vi "Create Evaluations.vi"(8 "error in (no error)":errorcluster, 11 "IEvaluation in":refnum<class "Null Adapter.lvclass">) -> (0 "error out":errorcluster, 2 "Evaluations Out":T1[](array[typedef]) {"Low Limit" format="%#_13g"; "SI Scaling" items=["femto"=-15, "pico"=-12, "nano"=-9, "micro"=-6, "milli"=-3, "percent"=-2, ""=0, "kilo"=3, "mega"=6, "giga"=9, "tera"=12]}, 3 "IEvaluation out":refnum<class "Null Adapter.lvclass">)   [LabVIEW 2018, in "SeqAuto Evaluations.lvlib" / "Null Adapter.lvclass"]
uses:
  Null Adapter.lvclass
  C:/Sequence Automation/Plugins/SeqAuto IEvaluation.lvlibp/SeqAuto IEvaluation.lvclass
  Plugins/TestStand API Tools (TSAT).lvlibp/Evaluation Actions/Includes/Controls/TSAT Evaluation.ctl
  Plugins/TestStand API Tools (TSAT).lvlibp/Evaluation Actions/Includes/Controls/TSAT Eval SI Unit Scaling.ctl
  Plugins/TestStand API Tools (TSAT).lvlibp/Evaluation Actions/Includes/Controls/TSAT Evaluation Type.ctl
  Plugins/SeqAuto IEvaluation.lvlibp/Read Measurement Name.vi
  Plugins/TestStand API Tools (TSAT).lvlibp/Evaluation Actions/TSAT Evaluation Actions.lvlib
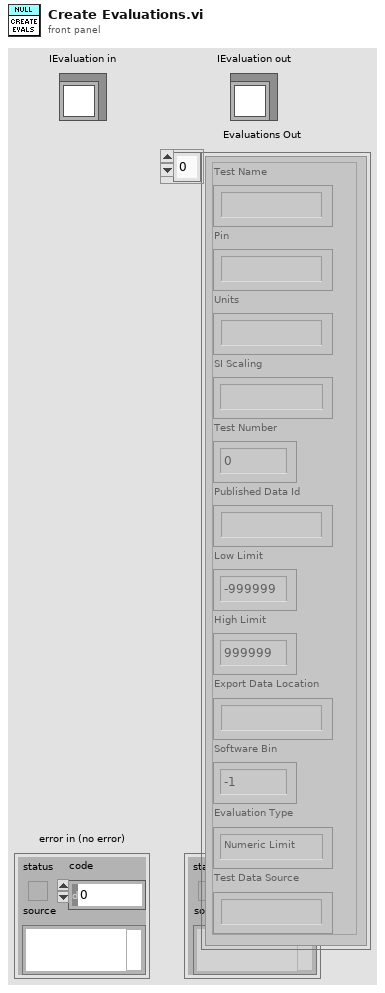
[diagram p1: front panel]
types:
  T1 = typedef "TestStand API Tools (TSAT).lvlibp/TSAT Evaluation Actions.lvlib/TSAT Evaluation.ctl" = cluster{"Test Name":string, "Pin":string, "Units":string, "SI Scaling":T2, "Test Number":i32, "Published Data Id":string, "Low Limit":dbl, "High Limit":dbl, "Export Data Location":string, "Software Bin":i64, "Evaluation Type":T3, "Test Data Source":string}
  T2 = typedef "TestStand API Tools (TSAT).lvlibp/TSAT Evaluation Actions.lvlib/TSAT Eval SI Unit Scaling.ctl" = i16
  T3 = typedef "TestStand API Tools (TSAT).lvlibp/TSAT Evaluation Actions.lvlib/TSAT Evaluation Type.ctl" = enum16{"Numeric Limit", "Pass/Fail", "None"}
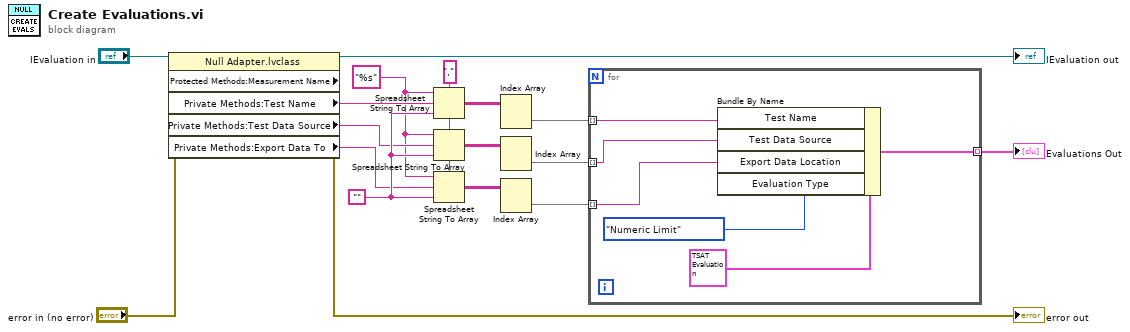
[diagram p0: block diagram]
diagram:
  w1 = "%s" ("format string")
  w10 = ""
  w11 = "," ("delimiter (Tab)")
  n1 = property class="Null Adapter.lvclass" props=["Protected Methods:Measurement Name", "Private Methods:Test Name", "Private Methods:Test Data Source", "Private Methods:Export Data To"](reference="IEvaluation in", error in="error in (no error)") -> (reference out=→"IEvaluation out":refnum<class "Null Adapter.lvclass">, error out=→"error out":errorcluster, "Private Methods:Test Name"=w12:string, "Private Methods:Test Data Source"=w2:string, "Private Methods:Export Data To"=w3:string)  [unwired: 1 out]
  n2 = Spreadsheet String To Array(delimiter (Tab)=w11, format string=w1, spreadsheet string=w12, array type (2D Dbl)=w10) -> (array=w9:string[][])
  n3 = Spreadsheet String To Array(delimiter (Tab)=w11, format string=w1, spreadsheet string=w2, array type (2D Dbl)=w10) -> (array=w7:string[][])
  n4 = Spreadsheet String To Array(delimiter (Tab)=w11, format string=w1, spreadsheet string=w3, array type (2D Dbl)=w10) -> (array=w5:string[][])
  n5 = Index Array(array=w9) -> (element=w8:string[])  [unwired: 2 in]
  n6 = Index Array(array=w7) -> (element=w6:string[])  [unwired: 2 in]
  n7 = Index Array(array=w5) -> (element=w4:string[])  [unwired: 2 in]
  n8 = for {
    tunnel: [w22] -> w13 mode=indexing
    tunnel: w8 -> [w20] mode=indexing
    tunnel: w6 -> [w19] mode=indexing
    tunnel: w4 -> [w18] mode=indexing
    n9 = Bundle By Name(cluster=T1 {"Test Name"="", "Pin"="", "Units"="", "SI Scaling"=0, "Test Number"=0, "Published Data Id"="", "Low Limit"=-999999.0, "High Limit"=999999.0, "Export Data Location"="", "Software Bin"=-1, "Evaluation Type"=enum."Numeric Limit", "Test Data Source"=""} ("Evaluation"), "Test Name"=w20, "Test Data Source"=w19, "Export Data Location"=w18, "Evaluation Type"=TSAT_Evaluation_Type."Numeric Limit") -> (w22:T1)
  }
  "Evaluations Out" <- w13
